vi "Get Window RefNum.vi"(6 "error in (no error)":errorcluster, 9 "window name (\"\")":string) -> (0 "error out":errorcluster, 3 "window refnum (NaWR)":T1)   [LabVIEW 2020, in "MacroAssert.lvlib" / "Win Util.lvlib"]
doc: "This VI will use the FindWindow API function to retrieve a window refnum for the window identified by window name. 'window name' is the text appearing in the title bar of a window. If the window cannot be found, the window refnum out will be 'Not a Window Refnum', and an error will occur."
uses:
  Win Util.lvlib
  Window Refnum.ctl
  user32.dll
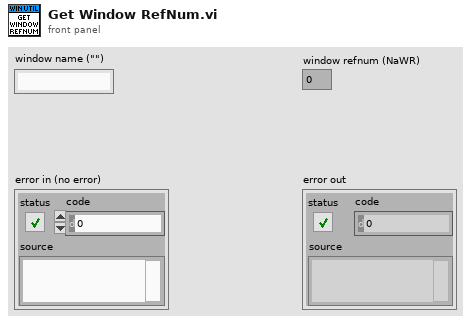
[diagram p1: front panel]
types:
  T1 = typedef "MacroAssert.lvlib/Win Util.lvlib/Window Refnum.ctl" = u64
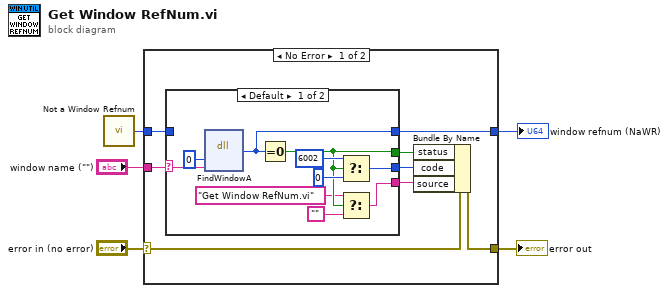
[diagram p0: block diagram]
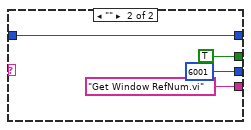
[diagram p2: hidden frame]
diagram:
  n1 = call "Not a Window Refnum.vi"() -> ("Not a Window Refnum"=w1:T1)
  n2 = case shown="No Error" "error in (no error)" {
    selector: "error in (no error)" -> [w10 w29]
    tunnel: [w12 w29] -> w5
    tunnel: [w11 w28] -> w2
    tunnel: "window name (\"\")" -> [w9 _]
    tunnel: w1 -> [w8 w28]
    frame No Error {
      n3 = case shown="Default" w9 {
        selector: w9 -> [w19 _]
        tunnel: [w23 w25] -> w11
        tunnel: [w17 TRUE] -> w13
        tunnel: [w22 6001] -> w7
        tunnel: w8 -> [_ w25]
        tunnel: [w15 "Get Window RefNum.vi"] -> w6
        frame Default {
          n4 = dll-call lib="user32.dll" fn="FindWindowA" label="FindWindow"("lpszClassName"=u64 0, "lpszWindowName"=w19) -> ("hWnd"=w23:u64)  [unwired: 5 in, 2 out]
          n5 = Equal To 0?(x=w23) -> (x = 0?=w17:bool)
          n6 = Select(t=6002, s=w17, f=0) -> (s? t:f=w22:i32)
          n7 = Select(t="Get Window RefNum.vi", s=w17, f="") -> (s? t:f=w15:string)
        }
        frame "" {
        }
      }
      n8 = Bundle By Name(cluster=w10, "status"=w13, "code"=w7, "source"=w6) -> (w12:errorcluster)
    }
    frame Error {
    }
  }
  "error out" <- w5
  "window refnum (NaWR)" <- w2
